vi "Close.vi"(8 "error in (no error)":errorcluster, 11 "PXI_MultiTrig in":refnum<class "PXI_MultiTrig.lvclass">) -> (0 "error out":errorcluster, 3 "PXI_MultiTrig out":refnum<class "PXI_MultiTrig.lvclass">)   [LabVIEW 2018, in "SyncPlugins.lvlib" / "PXI_MultiTrig.lvclass"]
uses:
  PXI_MultiTrig.lvclass
  X:/Projects/PMUCal/Modules/Sync/SyncPlugins/SyncPluginBase/SyncPluginBase.lvclass
  PXI_MultiTrig.lvclass/PXI_MultiTrig.ctl
  Typedefs/clClocks.ctl
  SyncPluginBase/SyncPluginBase.lvclass/SyncPluginBase.ctl
  Accessors/Read Triggers.vi
  Accessors/Read TimingSession.vi
  Accessors/Read RefClkSession.vi
  SyncPluginBase/Accessors/Read Initiated.vi
  Accessors/Read RefClkSource.vi
  Accessors/Write RefClkSession.vi
  Accessors/Write TimingSession.vi
  SyncPluginBase/Accessors/Write Initiated.vi
  SyncPluginBase/Accessors/Write Run.vi
  SyncPluginBase/Accessors/Write Locked.vi
  SyncPluginBase/Accessors/Read Clocks.vi
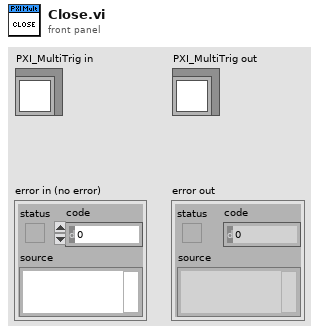
[diagram p1: front panel]
types:
  T1 = typedef "SyncPlugins.lvlib/PXI_MultiTrig.lvclass/clTrigger.ctl" = cluster{"Name":string, "DestTerm":string, "SrcTerm":string, "SyncClk":string, "Edge":i32, "Invert?":i32, "Initiated":bool, "Type":string, "TrigTime":bool}
  T2 = typedef "SyncPlugins.lvlib/PXI_MultiTrig.lvclass/clClocks.ctl" = cluster{"Name":string, "RefClk":string, "ClkTerminal":string, "Frequency":dbl, "DutyCycle":dbl, "ClkType":string, "Initiated":bool, "TrigTime":bool, "Delay":dbl}
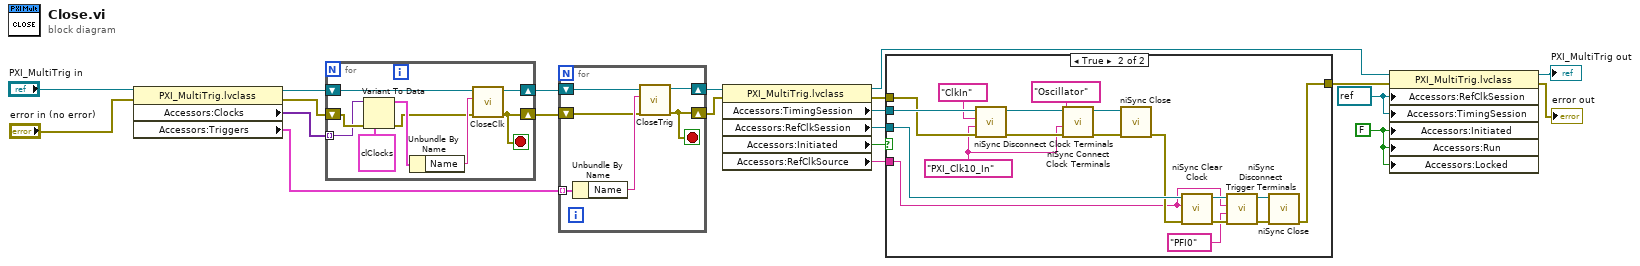
[diagram p0: block diagram]
diagram:
  w6 = refnum<k15> refnum ("RefClkSession")
  w7 = FALSE ("Initiated")
  n1 = property class="PXI_MultiTrig.lvclass"(reference="PXI_MultiTrig in", error in="error in (no error)") -> (reference out=w18:refnum<class "PXI_MultiTrig.lvclass">, error out=w17:errorcluster, "Accessors:Clocks"=w19:variant[], "Accessors:Triggers"=w14:T1[])
  n2 = for {
    tunnel: w19 -> [w25] mode=indexing
    shift-right: [w28] -> w16
    shift-left: w18 -> [w30]
    shift-right: [w27] -> w15
    shift-left: w17 -> [w26]
    stop <- w27 stop-if-true
    n3 = Variant To Data(error in=w26, type=T2 {"Name"="", "RefClk"="/PXI1Slot7/PFI1", "ClkTerminal"="PXI_Star4", "Frequency"=0.0, "DutyCycle"=0.0, "ClkType"="", "Initiated"=FALSE, "TrigTime"=FALSE, "Delay"=0.0} ("clClocks"), Variant=w25) -> (data=w24:T2, error out=w23:errorcluster)
    n4 = Unbundle By Name(w24) -> ("Name"=w29:string)
    n5 = call-dynamic "CloseClk.vi"("error in (no error)"=w23, "ClkName"=w29, "PXI_MultiTrig in"=w30) -> ("error out"=w27:errorcluster, "PXI_MultiTrig out"=w28:refnum<class "PXI_MultiTrig.lvclass">)  [unwired: 7 in]
  }
  n6 = for {
    shift-right: [w33] -> w13
    shift-left: w16 -> [w32]
    tunnel: w14 -> [w36] mode=indexing
    shift-right: [w31] -> w12
    shift-left: w15 -> [w34]
    stop <- w31 stop-if-true
    n7 = Unbundle By Name(w36) -> ("Name"=w35:string)
    n8 = call-dynamic "CloseTrig.vi"("error in (no error)"=w34, "TrigName"=w35, "PXI_MultiTrig in"=w32) -> ("error out"=w31:errorcluster, "PXI_MultiTrig out"=w33:refnum<class "PXI_MultiTrig.lvclass">)  [unwired: 7 in]
  }
  n9 = property class="PXI_MultiTrig.lvclass"(reference=w13, error in=w12) -> (reference out=w8:refnum<class "PXI_MultiTrig.lvclass">, error out=w10:errorcluster, "Accessors:TimingSession"=w11:refnum<k15>, "Accessors:RefClkSession"=w9:refnum<k15>, "Accessors:Initiated"=w2:bool, "Accessors:RefClkSource"=w1:string)
  n10 = case shown="True" w2 {
    tunnel: w11 -> [_ w55]
    tunnel: w10 -> [w37 w54]
    tunnel: w9 -> [_ w47]
    tunnel: [w37 w49] -> w5
    tunnel: w1 -> [_ w39]
    frame False {
    }
    frame True {
      w45 = "PXI_Clk10_In" ("destination terminal")
      n11 = call <instrlib>:"niSync Disconnect Clock Terminals.vi"("error in (no error)"=w54, "destination terminal"=w45, "source terminal"="ClkIn", "instrument handle"=w55) -> ("error out"=w53:errorcluster, "instrument handle out"=w52:refnum<k15>)  [unwired: 6 in]
      n12 = call <instrlib>:"niSync Connect Clock Terminals.vi"("error in (no error)"=w53, "destination terminal"=w45, "source terminal"="Oscillator", "instrument handle"=w52) -> ("error out"=w51:errorcluster, "instrument handle out"=w50:refnum<k15>)  [unwired: 6 in]
      n13 = call <instrlib>:"niSync Close.vi"("error in (no error)"=w51, "instrument handle"=w50) -> ("error out"=w46:errorcluster)  [unwired: 9 in]
      n14 = call <instrlib>:"niSync Clear Clock.vi"("error in (no error)"=w46, "terminal"=w39, "instrument handle"=w47) -> ("error out"=w41:errorcluster, "instrument handle out"=w43:refnum<k15>)  [unwired: 6 in]
      n15 = call <instrlib>:"niSync Disconnect Trigger Terminals.vi"("error in (no error)"=w41, "destination terminal"="PFI0", "source terminal"=w39, "instrument handle"=w43) -> ("error out"=w40:errorcluster, "instrument handle out"=w42:refnum<k15>)  [unwired: 6 in]
      n16 = call <instrlib>:"niSync Close.vi"("error in (no error)"=w40, "instrument handle"=w42) -> ("error out"=w49:errorcluster)  [unwired: 9 in]
    }
  }
  n17 = property class="PXI_MultiTrig.lvclass"(reference=w8, error in=w5, "Accessors:RefClkSession"=w6, "Accessors:TimingSession"=w6, "Accessors:Initiated"=w7, "Accessors:Run"=w7, "Accessors:Locked"=w7) -> (reference out=→"PXI_MultiTrig out":refnum<class "PXI_MultiTrig.lvclass">, error out=→"error out":errorcluster)
